vi "SendMessage.vi"(4 "Value":string, 5 "Name":string, 6 "error in":errorcluster, 7 "timeout in ms (-1)":i32, 9 "message queue in":T1) -> (0 "error out":errorcluster, 1 "timed out?":bool, 3 "message queue out":T1)   [LabVIEW 2014, in "Raspberry Pi Compatible Compiler for LabVIEW.lvlib" / "SimpleMessaging.lvlib"]
uses:
  SimpleMessaging.lvlib
  MessageQueueTD.ctl
  MessageTD.ctl
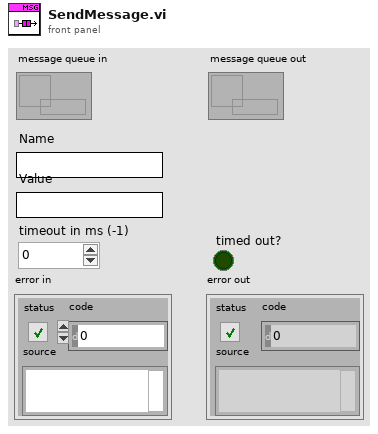
[diagram p1: front panel]
types:
  T1 = typedef "Raspberry Pi Compatible Compiler for LabVIEW.lvlib/SimpleMessaging.lvlib/MessageQueueTD.ctl" = refnum<queue>
  T2 = typedef "Raspberry Pi Compatible Compiler for LabVIEW.lvlib/SimpleMessaging.lvlib/MessageTD.ctl" = cluster{"Name":string, "Value":string}
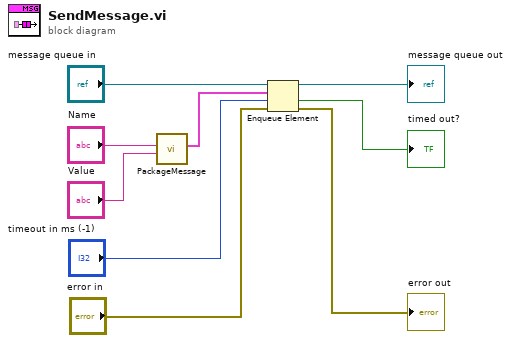
[diagram p0: block diagram]
diagram:
  n1 = call "PackageMessage.vi"("Value"="Value", "Name"="Name") -> ("Message"=w6:T2)  [unwired: 9 in]
  n2 = Enqueue Element(queue="message queue in", element=w6, timeout in ms (-1)="timeout in ms (-1)", error in (no error)="error in") -> (queue out=→"message queue out":T1, timed out?=→"timed out?":bool, error out=→"error out":errorcluster)
